vi "ScopeInit.vi"(1 "error in (no error)":errorcluster) -> (0 "error out":errorcluster)   [LabVIEW 2012]
uses:
  Program Files (x86)/National Instruments/LabVIEW 2018/instr.lib/Tektronix DPO MSO 2000 4000 Series/Tektronix DPO MSO 2000 4000 Series.lvlib
  Program Files (x86)/National Instruments/LabVIEW 2018/instr.lib/Tektronix DPO MSO 2000 4000 Series/Public/Configure/Configure Trigger (Edge).vi
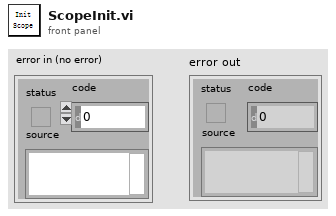
[diagram p1: front panel]
types:
  T1 = typedef "IMAQ Image.ctl" = refnum<image>
  T2 = cluster{"示波器":cluster{"Channel (0:Channel 1)":enum16{"Channel 1", "Channel 2", "Channel 3", "Channel 4"}, "电压范围":dbl, "触发电压":dbl, "时间范围":dbl, " 示波器VISA":refnum<visa-resource-name>}, "光谱仪":cluster{"Channel (0:Channel 1)":enum16{"Channel 1", "Channel 2", "Channel 3", "Channel 4"}, "电压范围":u64, "触发电压":u64, "时间范围":u64}, " 相机1":cluster{"曝光时间":i32, "模拟增益":i32, "控制套接字":i32, "IP 地址":string, " 采集套接字":i32, "  版本号":i32, "ImageData":T1, "  增益最大":i32, "  增益最小":i32, " 曝光最大":i32, " 曝光最小":i32, " 帧速":i32, " 同步切换":i32, "  曝光缩放":i32}, " 偏振仪":cluster{"波长范围":enum16{"可见光", "近红外"}, "电压范围":u64, "触发电压":u64, "时间范围":u64}, " 功率计":cluster{"通道":enum16{"Channel 1", "Channel 2"}, "工作波长":u64, "单位":u64, "时间范围":u64}, "能量计":cluster{"通道":enum16{"Channel 1", "Channel 2"}, "工作波长":u64, "单位":u64, "时间范围":u64}, "电机":cluster{"Channel (0:Channel 1)":enum16{"Channel 1", "Channel 2", "Channel 3", "Channel 4"}, "电压范围":u64, "触发电压":u64, "时间范围":u64}}
  T3 = cluster{"Channel (0:Channel 1)":enum16{"Channel 1", "Channel 2", "Channel 3", "Channel 4"}, "电压范围":dbl, "触发电压":dbl, "时间范围":dbl, " 示波器VISA":refnum<visa-resource-name>}
  T4 = enum16{"Channel 1", "Channel 2", "Channel 3", "Channel 4"}
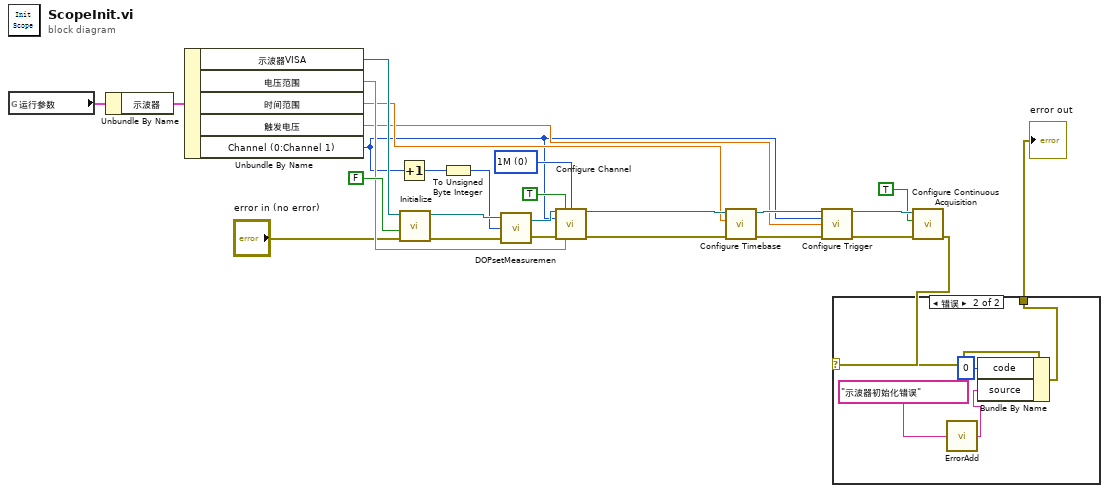
[diagram p0: block diagram]
diagram:
  w18 = u16 0 items=["1M", "75", "50"] ("Input Impedance (0: 1M ohm)")
  n1 = global read "参数.vi" "运行参数"() -> (w10:T2)
  n2 = Unbundle By Name(w10) -> ("示波器"=w9:T3)
  n3 = Unbundle By Name(w9) -> ("示波器VISA"=w8:refnum<visa-resource-name>, "电压范围"=w7:dbl, "时间范围"=w6:dbl, "触发电压"=w5:dbl, "Channel (0:Channel 1)"=w3:T4)
  n4 = Increment(x=w3) -> (x+1=w23:T4)
  n5 = call "Initialize.vi"("error in (no error)"="error in (no error)", "Reset (True)"=FALSE, "VISA resource name"=w8) -> ("error out"=w24:errorcluster, "VISA resource name out"=w25:refnum<visa-resource-name>)  [unwired: 7 in]
  n6 = To Unsigned Byte Integer(number=w23) -> (unsigned 8bit integer=w22:u8)
  n7 = call "DOPsetMeasuremen.vi"("error in (no error)"=w24, "CH"=w22, "VISA resource name"=w25) -> ("error out"=w20:errorcluster, "VISA resource name out"=w21:refnum<visa-resource-name>)
  n8 = call "Configure Channel.vi"("VISA resource name"=w21, "Enable Channel (T: Enable)"=TRUE, "Input Impedance (0: 1M ohm)"=w18, "Channel (0: Channel 1)"=w3, "error in (no error)"=w20, "Vertical Range (10.0 V)"=w7) -> ("VISA resource name out"=w17:refnum<visa-resource-name>, "error out"=w16:errorcluster)  [unwired: 8 in]
  n9 = call "Configure Timebase.vi"("error in (no error)"=w16, "Timebase (0.0005 s)"=w6, "VISA resource name"=w17) -> ("error out"=w14:errorcluster, "VISA resource name out"=w15:refnum<visa-resource-name>)  [unwired: 7 in]
  n10 = call-poly "Configure Trigger.vi"("VISA resource name"=w15, "Trigger Source (0: Channel 1)"=w3, "Trigger Level (0.0 V)"=w5, "error in (no error)"=w14) -> ("VISA resource name out"=w13:refnum<visa-resource-name>, "error out"=w12:errorcluster)  [unwired: 10 in]
  n11 = call "Configure Continuous Acquisition.vi"("error in (no error)"=w12, "Enable Continuous Acquisition Mode (T: Enable)"=TRUE, "VISA resource name"=w13) -> ("error out"=w2:errorcluster)  [unwired: 7 in, 1 out]
  n12 = case shown="错误" w2 {
    selector: w2 -> [w27 w32]
    tunnel: [w27 w30] -> w1
    frame No Error {
    }
    frame Error {
      n13 = call "ErrorAdd.vi"("source"="示波器初始化错误") -> ("Errorout Souce"=w28:string)
      n14 = Bundle By Name(cluster=w32, "code"=0, "source"=w28) -> (w30:errorcluster)
    }
  }
  "error out" <- w1
